vi "MoveRecordScroll.vi"(9 "Scroll Value":u8, 10 "Direction":enum16{"Up", "Down"}(ring), 11 "ArrayRef":refnum<vi>) -> ()   [LabVIEW 2018, in "Library-Ctrl.lvlib"]
uses:
  Library-Ctrl.lvlib
  <vilib>/Utility/miscctls.llb/LVRowAndColumnUnsignedTypeDef.ctl
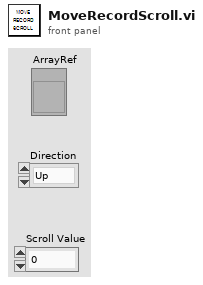
[diagram p1: front panel]
types:
  T1 = typedef "LVRowAndColumnUnsignedTypeDef.ctl" = cluster{"Row":u32, "Column":u32}
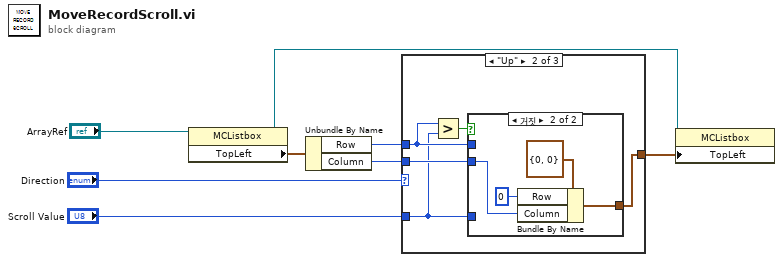
[diagram p0: block diagram]
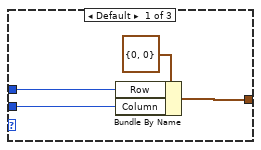
[diagram p2: hidden frame]
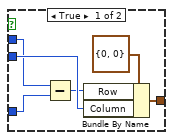
[diagram p3: hidden frame]
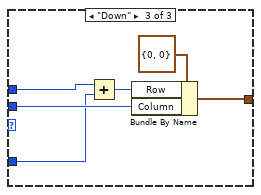
[diagram p4: hidden frame]
diagram:
  n1 = property class="MCListbox"(reference="ArrayRef") -> (reference out=w2:refnum<vi>, "TopLeft"=w7:T1)  [unwired: 1 in, 1 out]
  n2 = Unbundle By Name(w7) -> ("Row"=w5:u32, "Column"=w4:u32)
  n3 = case shown="\"Up\"" "Direction" {
    tunnel: w5 -> [w11 w14 w30]
    tunnel: w4 -> [w10 w17 w32]
    tunnel: "Scroll Value" -> [_ w13 w29]
    tunnel: [w9 w16 w28] -> w1
    frame Default {
      n4 = Bundle By Name(cluster=T1 {"Row"=0, "Column"=0} ("인덱스 값"), "Row"=w11, "Column"=w10) -> (w9:T1)
    }
    frame "Up" {
      n5 = Greater?(x=w14, y=w13) -> (0:w15:bool)
      n6 = case shown="거짓" w15 {
        tunnel: w17 -> [w22 w26]
        tunnel: w13 -> [w19 _]
        tunnel: [w20 w25] -> w16
        tunnel: w14 -> [w18 _]
        frame True {
          n7 = Subtract(x=w18, y=w19) -> (x-y=w21:u32)
          n8 = Bundle By Name(cluster=T1 {"Row"=0, "Column"=0} ("인덱스 값"), "Row"=w21, "Column"=w22) -> (w20:T1)
        }
        frame False {
          n9 = Bundle By Name(cluster=T1 {"Row"=0, "Column"=0} ("인덱스 값"), "Row"=u32 0, "Column"=w26) -> (w25:T1)
        }
      }
    }
    frame "Down" {
      n10 = Add(x=w30, y=w29) -> (x+y=w31:u32)
      n11 = Bundle By Name(cluster=T1 {"Row"=0, "Column"=0} ("인덱스 값"), "Row"=w31, "Column"=w32) -> (w28:T1)
    }
  }
  n12 = property class="MCListbox"(reference=w2, "TopLeft"=w1) -> ()  [unwired: 1 in, 2 out]
